vi "Avantes - plot.vi"(8 "error in (no error)":errorcluster, 9 "notifier":refnum<notifier>, 10 "Output Ready":i32, 11 "Cluster in":T1) -> (0 "error out":errorcluster, 2 "a_pTimeLabel1":u32, 3 "Scope Values":cluster{"Y":dbl[], "Y":dbl[]}[](graph))   [LabVIEW 2013, in "Avantes Spectrometer Functions.lvlib"]
uses:
  Avantes Spectrometer Functions.lvlib
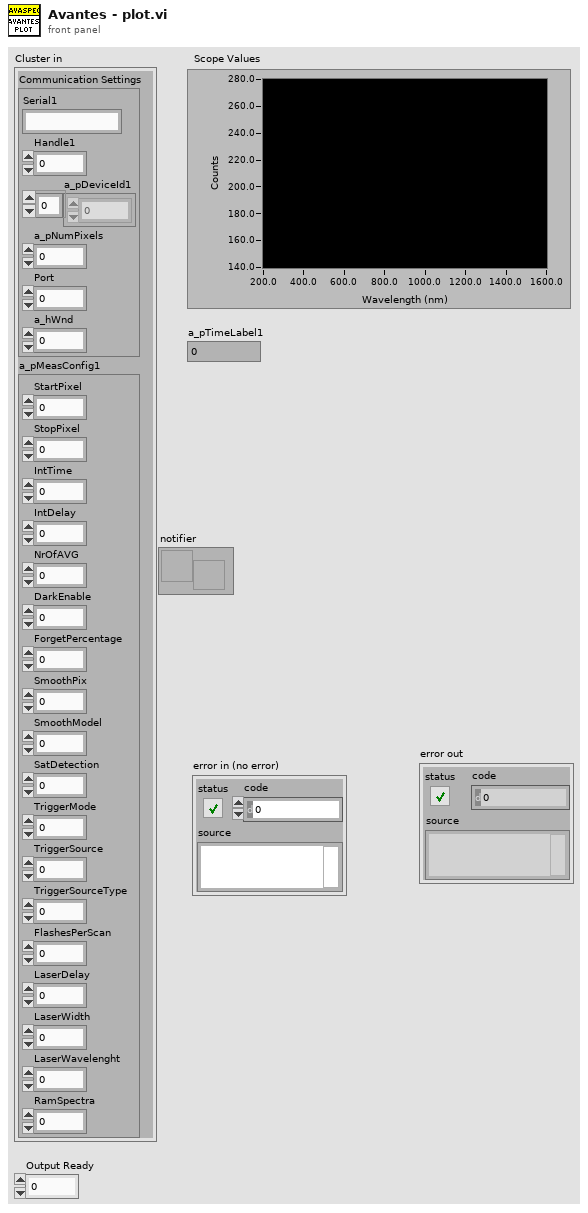
[diagram p1: front panel]
types:
  T1 = cluster{"Communication Settings":cluster{"Serial1":string, "Handle1":i32, "a_pDeviceId1":u8[], "a_pNumPixels":u16, "Port":i32, "a_hWnd":i32}, "a_pMeasConfig1":cluster{"StartPixel":u16, "StopPixel":u16, "IntTime":sgl, "IntDelay":u32, "NrOfAVG":u32, "DarkEnable":u8, "ForgetPercentage":u8, "SmoothPix":u16, "SmoothModel":u8, "SatDetection":u8, "TriggerMode":u8, "TriggerSource":u8, "TriggerSourceType":u8, "FlashesPerScan":u16, "LaserDelay":u32, "LaserWidth":u32, "LaserWavelenght":sgl, "RamSpectra":u16}}
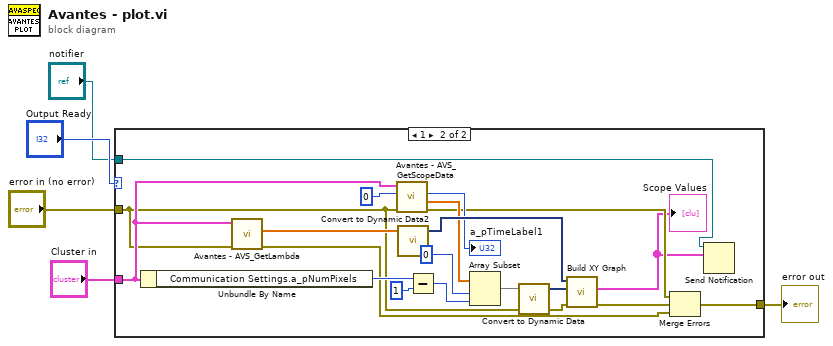
[diagram p0: block diagram]
diagram:
  n1 = case shown="1" "Output Ready" {
    tunnel: "Cluster in" -> [_ w14]
    tunnel: "error in (no error)" -> [w6 w13]
    tunnel: [w6 w9] -> w3
    tunnel: "notifier" -> [_ w8]
    frame 0, Default {
    }
    frame 1 {
      n2 = Unbundle By Name(w14) -> ("Communication Settings.a_pNumPixels"=w15:u16)
      n3 = call "Avantes - AVS_GetLambda.vi"("error in (no error)"=w13, "Cluster in"=w14) -> ("error out"=w11:errorcluster, "a_pWaveLength"=w16:dbl[])  [unwired: 7 in, 1 out]
      n4 = call "Avantes - AVS_GetScopeData.vi"("error in (no error)"=w13, "a_pTimeLabel"=0, "Cluster in"=w14) -> ("error out"=w10:errorcluster, "a_pSpectrum"=w18:dbl[], "a_pTimeLabel 2"=→"a_pTimeLabel1":u32)  [unwired: 5 in, 1 out]
      n5 = call "Convert to Dynamic Data2"("Array"=w16) -> ("Dynamic Data Type"=w24:dynamicdata)  [unwired: 3 in]
      n6 = Subtract(x=w15, y=u16 1) -> (x-y=w22:u16)
      n7 = Array Subset(array=w18, index=0, length=w22) -> (w20:dbl[])
      n8 = call "Convert to Dynamic Data"("Array"=w20) -> ("Dynamic Data Type"=w25:dynamicdata)  [unwired: 3 in]
      n9 = call "Build XY Graph"("error in (no error)"=w13, "Y Input"=w25, "X Input"=w24) -> ("error out"=w12:errorcluster, "XY Graph"=w7:cluster{"Y":dbl[], "Y":dbl[]}[])  [unwired: 7 in]
      "Scope Values" <- w7
      n10 = Merge Errors(w10, w12, w11) -> (w9:errorcluster)
      n11 = Send Notification(notification=w7, notifier=w8) -> ()  [unwired: 1 in, 2 out]
    }
  }
  "error out" <- w3
